vi "Meacurrent.vi"(8 "error in":errorcluster caption="错误输入（无错误）", 10 "测试类型":u16(ring) items=["DCV", "ACV", "DCI", "ACI", "OHM", "RST", "CAP", "FRQ", "AUTO"], 11 "VISA":refnum<visa-resource-name>="COM1") -> (0 "error out":errorcluster caption="错误输出", 2 "数值":dbl format="%#_3g")   [LabVIEW 2013]
uses:
  C:/Program Files/National Instruments/LabVIEW 2013/examples/Instrument IO/Serial/support/Serial - Settings.ctl
  <vilib>/Instr/_visa.llb/VISA Configure Serial Port (Instr).vi
panel:
  out "响应":string
  in  "串口设置":T1={"波特率"=9600, "数据比特"=8, "奇偶"=enum."None", "停止位"=10, "流控制"=0} {"流控制" items=["无"=0, "XON/XOFF"=1, "RTS/CTS"=2, "DTR/DSR"=4]; "停止位" items=["1.0"=10, "1.5"=15, "2.0"=20]; "数据比特" min=5 max=8 step=1; "波特率" items=["75"=75, "110"=110, "134"=134, "150"=150, "300"=300, "600"=600, "1200"=1200, "1800"=1800, "2400"=2400, "4800"=4800, "7200"=7200, "9600"=9600, "14400"=14400, "19200"=19200, "28800"=28800, "38400"=38400, "56000"=56000, "57600"=57600, "115200"=115200, "128000"=128000, "230400"=230400]}
  in  "读取前延时(ms)":u32=600
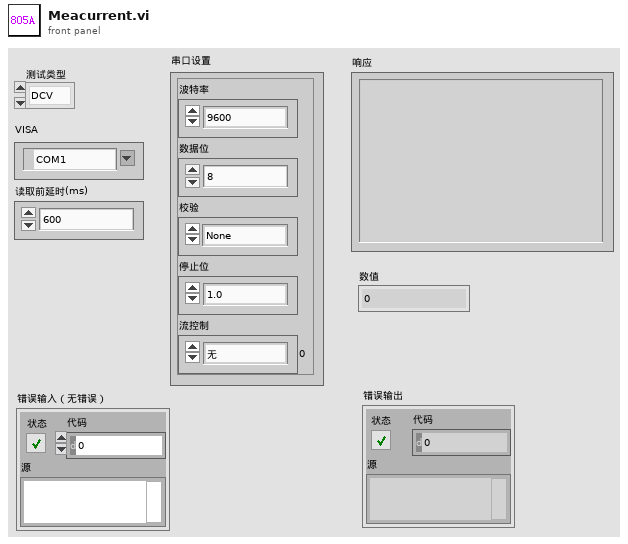
[diagram p1: front panel]
types:
  T1 = typedef "Serial - Settings.ctl" = cluster{"波特率":u32, "数据比特":u16, "奇偶":enum16{"None", "Odd", "Even", "Mark", "Space"}, "停止位":u16, "流控制":u16}
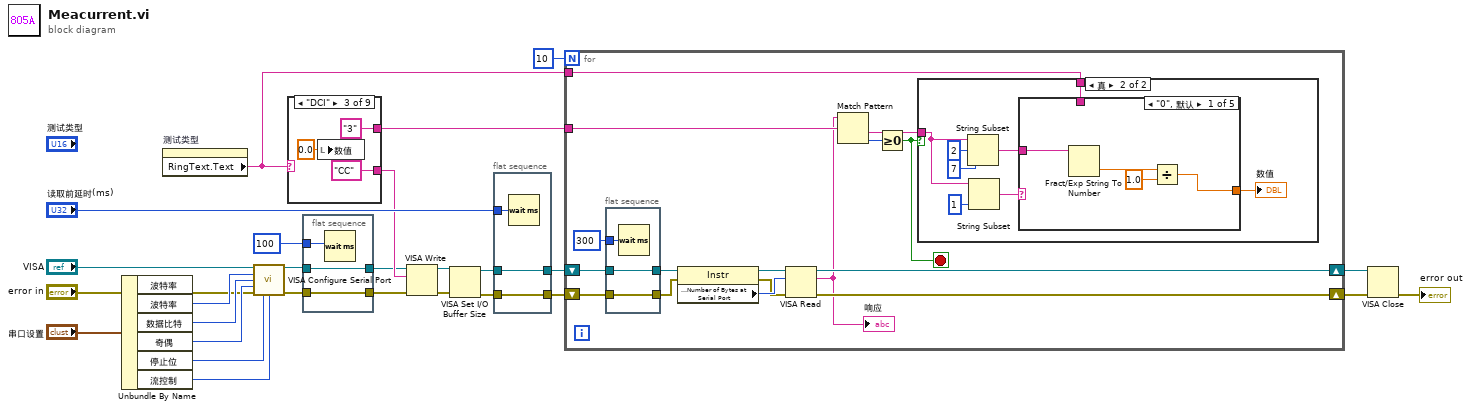
[diagram p0: block diagram]
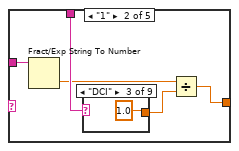
[diagram p3: hidden frame]
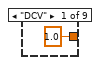
[diagram p4: hidden frame]
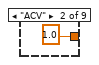
[diagram p5: hidden frame]
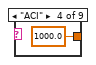
[diagram p6: hidden frame]
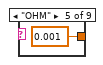
[diagram p7: hidden frame]
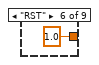
[diagram p8: hidden frame]
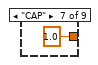
[diagram p9: hidden frame]
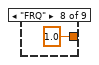
[diagram p10: hidden frame]
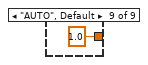
[diagram p11: hidden frame]
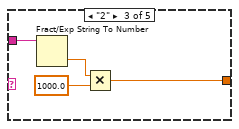
[diagram p12: hidden frame]
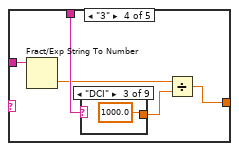
[diagram p13: hidden frame]
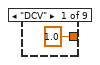
[diagram p14: hidden frame]
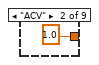
[diagram p15: hidden frame]
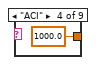
[diagram p16: hidden frame]
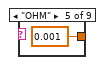
[diagram p17: hidden frame]
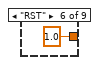
[diagram p18: hidden frame]
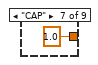
[diagram p19: hidden frame]
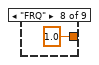
[diagram p20: hidden frame]
diagram:
  n1 = Unbundle By Name("串口设置") -> ("波特率"=w20:u32, "数据比特"=w19:u16, "奇偶"=w18:enum16{"None", "Odd", "Even", "Mark", "Space"}, "停止位"=w17:u16, "流控制"=w16:u16)  [unwired: 1 out]
  n2 = property on="测试类型" class="Ring (严格)"() -> ("RingText.Text"=w3:string)  [unwired: 2 in, 2 out]
  n3 = call-poly "VISA Configure Serial Port"("VISA resource name"="VISA", "baud rate (9600)"=w20, "data bits (8)"=w19, "parity (0:none)"=w18, "error in (no error)"="error in", "stop bits (10: 1 bit)"=w17, "flow control (0:none)"=w16) -> ("VISA resource name out"=w12:refnum<visa-resource-name>, "error out"=w11:errorcluster)  [unwired: 2 in, 5 out]
  n4 = case shown="\"DCI\"" w3 {
    tunnel: ["AA" ("Command") "BB" ("Command") "CC" ("Command") "DD" ("Command") "EE" ("Command") "FF" ("Command") "GG" ("Command") "HH" ("Command") "MM" ("Command")] -> w15
    tunnel: ["0" ("Command") "1" ("Command") "3" ("Command") "4" ("Command") "6" ("Command") "F" ("Command") "7" ("Command") "8" ("Command") "M" ("Command")] -> w14
    frame "DCV" {
    }
    frame "ACV" {
    }
    frame "DCI" {
      n5 = local write "数值"(0.0 ("数值")) -> ()
    }
    frame "ACI" {
    }
    frame "OHM" {
    }
    frame "RST" {
    }
    frame "CAP" {
    }
    frame "FRQ" {
    }
    frame "AUTO", Default {
    }
  }
  n6 = flat-sequence {
    tunnel: w11 -> [w49]
    tunnel: [w49] -> w10
    tunnel: [w48] -> w9
    tunnel: w12 -> [w48]
    tunnel: u32 100 ("读取前延时(ms)") -> [w47]
    frame #0 {
      n7 = Wait (ms)(milliseconds to wait=w47) -> ()  [unwired: 1 out]
    }
  }
  n8 = VISA Write(VISA resource name=w9, write buffer=w15, error in (no error)=w10) -> (VISA resource name out=w6:refnum<visa-resource-name>, error out=w7:errorcluster)  [unwired: 1 out]
  n9 = VISA Set I/O Buffer Size(VISA resource name=w6, error in (no error)=w7) -> (VISA resource name out=w5:refnum<visa-resource-name>, error out=w4:errorcluster)  [unwired: 2 in]
  n10 = flat-sequence {
    tunnel: w4 -> [w50]
    tunnel: [w50] -> w24
    tunnel: [w51] -> w23
    tunnel: "读取前延时(ms)" -> [w52]
    tunnel: w5 -> [w51]
    frame #0 {
      n11 = Wait (ms)(milliseconds to wait=w52) -> ()  [unwired: 1 out]
    }
  }
  n12 = for {
    N: 10 -> [_]
    tunnel: w14 -> [w65]
    shift-right: [w67] -> w25
    shift-left: w23 -> [w61]
    shift-right: [w68] -> w26
    shift-left: w24 -> [w59]
    tunnel: w3 -> [w53]
    stop <- w56 stop-if-true
    n13 = flat-sequence {
      tunnel: w59 -> [w70]
      tunnel: [w70] -> w58
      tunnel: w61 -> [w69]
      tunnel: [w69] -> w60
      tunnel: u32 300 ("读取前延时(ms)") -> [w71]
      frame #0 {
        n14 = Wait (ms)(milliseconds to wait=w71) -> ()  [unwired: 1 out]
      }
    }
    n15 = property class="Instr"(reference=w60, error in=w58) -> (reference out=w55:refnum<visa-resource-name>, error out=w54:errorcluster, "Serial Settings:Number of Bytes at Serial Port"=w66:u32)
    n16 = VISA Read(VISA resource name=w55, byte count=w66, error in (no error)=w54) -> (VISA resource name out=w67:refnum<visa-resource-name>, read buffer=w62:string, error out=w68:errorcluster)  [unwired: 1 out]
    "响应" <- w62
    n17 = Match Pattern(string=w62, regular expression=w65) -> (after substring=w63:string, offset past match=w64:i32)  [unwired: 1 in, 2 out]
    n18 = Greater Or Equal To 0?(x=w64) -> (x >= 0?=w56:bool)
    n19 = case shown="真" w56 {
      tunnel: w63 -> [_ w77]
      tunnel: w53 -> [_ w73]
      frame False {
      }
      frame True {
        n20 = String Subset(string=w77, offset (0)=2 ("偏移量(0)"), length (rest)=7 ("长度（剩余）")) -> (substring=w74:string)
        n21 = String Subset(string=w77, length (rest)=1 ("长度（剩余）")) -> (substring=w78:string)  [unwired: 1 in]
        n22 = case shown="\"0\", 默认" w78 {
          tunnel: w74 -> [w83 w88 w101 w106 w120]
          tunnel: w73 -> [_ w87 _ w105 w119]
          tunnel: [w81 w84 w98 w102 w116] -> w72
          frame "0", Default {
            n23 = Fract/Exp String To Number(string=w83) -> (number=w82:dbl)  [unwired: 3 in, 1 out]
            n24 = Divide(x=w82, y=1.0 ("数字")) -> (x/y=w81:dbl)
          }
          frame "1" {
            n25 = Fract/Exp String To Number(string=w88) -> (number=w86:dbl)  [unwired: 3 in, 1 out]
            n26 = case shown="\"DCI\"" w87 {
              tunnel: [1.0 1.0 1.0 1000.0 0.001 1.0 1.0 1.0 1.0] -> w85
              frame "DCV" {
              }
              frame "ACV" {
              }
              frame "DCI" {
              }
              frame "ACI" {
              }
              frame "OHM" {
              }
              frame "RST" {
              }
              frame "CAP" {
              }
              frame "FRQ" {
              }
              frame "AUTO", Default {
              }
            }
            n27 = Divide(x=w86, y=w85) -> (x/y=w84:dbl)
          }
          frame "2" {
            n28 = Fract/Exp String To Number(string=w101) -> (number=w100:dbl)  [unwired: 3 in, 1 out]
            n29 = Multiply(x=w100, y=1000.0) -> (x*y=w98:dbl)
          }
          frame "3" {
            n30 = Fract/Exp String To Number(string=w106) -> (number=w104:dbl)  [unwired: 3 in, 1 out]
            n31 = case shown="\"DCI\"" w105 {
              tunnel: [1.0 1.0 1000.0 1000.0 0.001 1.0 1.0 1.0 1.0] -> w103
              frame "DCV" {
              }
              frame "ACV" {
              }
              frame "DCI" {
              }
              frame "ACI" {
              }
              frame "OHM" {
              }
              frame "RST" {
              }
              frame "CAP" {
              }
              frame "FRQ" {
              }
              frame "AUTO", Default {
              }
            }
            n32 = Divide(x=w104, y=w103) -> (x/y=w102:dbl)
          }
          frame "4" {
            n33 = Fract/Exp String To Number(string=w120) -> (number=w118:dbl)  [unwired: 3 in, 1 out]
            n34 = case shown="\"DCI\"" w119 {
              tunnel: [1.0 1.0 1000.0 1000.0 1e-06 1.0 1.0 1.0 1.0] -> w117
              frame "DCV" {
              }
              frame "ACV" {
              }
              frame "DCI" {
              }
              frame "ACI" {
              }
              frame "OHM" {
              }
              frame "RST" {
              }
              frame "CAP" {
              }
              frame "FRQ" {
              }
              frame "AUTO", Default {
              }
            }
            n35 = Divide(x=w118, y=w117) -> (x/y=w116:dbl)
          }
        }
        "数值" <- w72
      }
    }
  }
  n36 = VISA Close(VISA resource name=w25, error in (no error)=w26) -> (error out=→"error out":errorcluster)
